vi "Relays1.vi"() -> ()   [LabVIEW 2011]
uses:
  low_level_proc/relaySpec.ctl
panel:
  out "P Run":T1={"Card Index"=2, "Relay Index"=4} {"Card Index" items=["1", "2", "3", "4", "5"]; "Relay Index" items=["1", "2", "3", "4", "5", "6", "7", "8", "9", "10", "11", "12"]}
  out "P H2 Flush":T1={"Card Index"=2, "Relay Index"=3} {"Card Index" items=["1", "2", "3", "4", "5"]; "Relay Index" items=["1", "2", "3", "4", "5", "6", "7", "8", "9", "10", "11", "12"]}
  out "P In":T1={"Card Index"=2, "Relay Index"=2} {"Card Index" items=["1", "2", "3", "4", "5"]; "Relay Index" items=["1", "2", "3", "4", "5", "6", "7", "8", "9", "10", "11", "12"]}
  out "P Active":T1={"Card Index"=2, "Relay Index"=1} {"Card Index" items=["1", "2", "3", "4", "5"]; "Relay Index" items=["1", "2", "3", "4", "5", "6", "7", "8", "9", "10", "11", "12"]}
  out "P Remote":T1={"Card Index"=2, "Relay Index"=0} {"Card Index" items=["1", "2", "3", "4", "5"]; "Relay Index" items=["1", "2", "3", "4", "5", "6", "7", "8", "9", "10", "11", "12"]}
  out "In Run":T1={"Card Index"=0, "Relay Index"=10} {"Card Index" items=["1", "2", "3", "4", "5"]; "Relay Index" items=["1", "2", "3", "4", "5", "6", "7", "8", "9", "10", "11", "12"]}
  out "In Bubbler In":T1={"Card Index"=0, "Relay Index"=9} {"Card Index" items=["1", "2", "3", "4", "5"]; "Relay Index" items=["1", "2", "3", "4", "5", "6", "7", "8", "9", "10", "11", "12"]}
  out "In Active":T1={"Card Index"=0, "Relay Index"=8} {"Card Index" items=["1", "2", "3", "4", "5"]; "Relay Index" items=["1", "2", "3", "4", "5", "6", "7", "8", "9", "10", "11", "12"]}
  out "In Remote":T1={"Card Index"=0, "Relay Index"=7} {"Card Index" items=["1", "2", "3", "4", "5"]; "Relay Index" items=["1", "2", "3", "4", "5", "6", "7", "8", "9", "10", "11", "12"]}
  out "Al Run":T1={"Card Index"=0, "Relay Index"=6} {"Card Index" items=["1", "2", "3", "4", "5"]; "Relay Index" items=["1", "2", "3", "4", "5", "6", "7", "8", "9", "10", "11", "12"]}
  out "Al Bubbler In":T1={"Card Index"=0, "Relay Index"=5} {"Card Index" items=["1", "2", "3", "4", "5"]; "Relay Index" items=["1", "2", "3", "4", "5", "6", "7", "8", "9", "10", "11", "12"]}
  out "Al Active":T1={"Card Index"=0, "Relay Index"=4} {"Card Index" items=["1", "2", "3", "4", "5"]; "Relay Index" items=["1", "2", "3", "4", "5", "6", "7", "8", "9", "10", "11", "12"]}
  out "Al Remote":T1={"Card Index"=0, "Relay Index"=3} {"Card Index" items=["1", "2", "3", "4", "5"]; "Relay Index" items=["1", "2", "3", "4", "5", "6", "7", "8", "9", "10", "11", "12"]}
  out "Ga H2 Dilute":T1={"Card Index"=3, "Relay Index"=4} {"Card Index" items=["1", "2", "3", "4", "5"]; "Relay Index" items=["1", "2", "3", "4", "5", "6", "7", "8", "9", "10", "11", "12"]}
  out "Ga Run":T1={"Card Index"=3, "Relay Index"=3} {"Card Index" items=["1", "2", "3", "4", "5"]; "Relay Index" items=["1", "2", "3", "4", "5", "6", "7", "8", "9", "10", "11", "12"]}
  out "Ga Bubbler In":T1={"Card Index"=3, "Relay Index"=2} {"Card Index" items=["1", "2", "3", "4", "5"]; "Relay Index" items=["1", "2", "3", "4", "5", "6", "7", "8", "9", "10", "11", "12"]}
  out "Ga Active":T1={"Card Index"=3, "Relay Index"=1} {"Card Index" items=["1", "2", "3", "4", "5"]; "Relay Index" items=["1", "2", "3", "4", "5", "6", "7", "8", "9", "10", "11", "12"]}
  out "Ga Remote":T1={"Card Index"=3, "Relay Index"=0} {"Card Index" items=["1", "2", "3", "4", "5"]; "Relay Index" items=["1", "2", "3", "4", "5", "6", "7", "8", "9", "10", "11", "12"]}
  # "Relay Card #"
  # "Relay #"
  # "Relay Card #"
  # "Relay #"
  # "Relay Card #"
  # "Relay #"
  # "Relay Card #"
  # "Relay #"
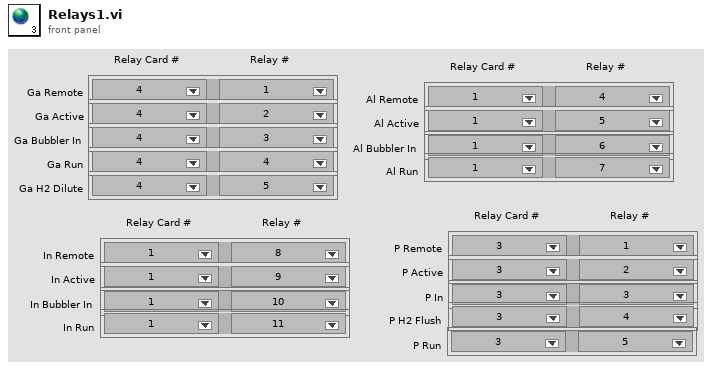
[diagram p1: front panel]
types:
  T1 = typedef "relaySpec.ctl" = cluster{"Card Index":u16, "Relay Index":u16}
diagram:
